vi "Receiver_Example.vi"() -> ()   [LabVIEW 2014]
panel:
  out "created new?":bool
  out "XY Graph":cdb[](graph)
  out "Modulation parameter":T1
  out "string 2":string
  out "SIG valid?":bool
  out "Frequency offset":dbl
  in  "stop":bool
  out "USRP CoercedParamters":T2={"coerced IQ rate"=100000.0, "coerced carrier frequency"=100000.0, "coerced gain"=0.0} {"coerced gain" format="%#_6f"; "coerced carrier frequency" format="%#_6p"; "coerced IQ rate" format="%#_6p"}
  out "error out":errorcluster
  in  "Trigger level":dbl=0.005 format="%f"
  in  "error in (no error)":errorcluster
  in  "USRP ControledParameters":T3={"active antenna"="RX2", "gain"=20.0, "carrier frequency"=5800000000.0, "IQ rate"=2000000.0} {"IQ rate" format="%#_6p"; "carrier frequency" format="%#_6p"; "gain" format="%#_6f"}
  in  "device names":refnum<k15>="NI2900"
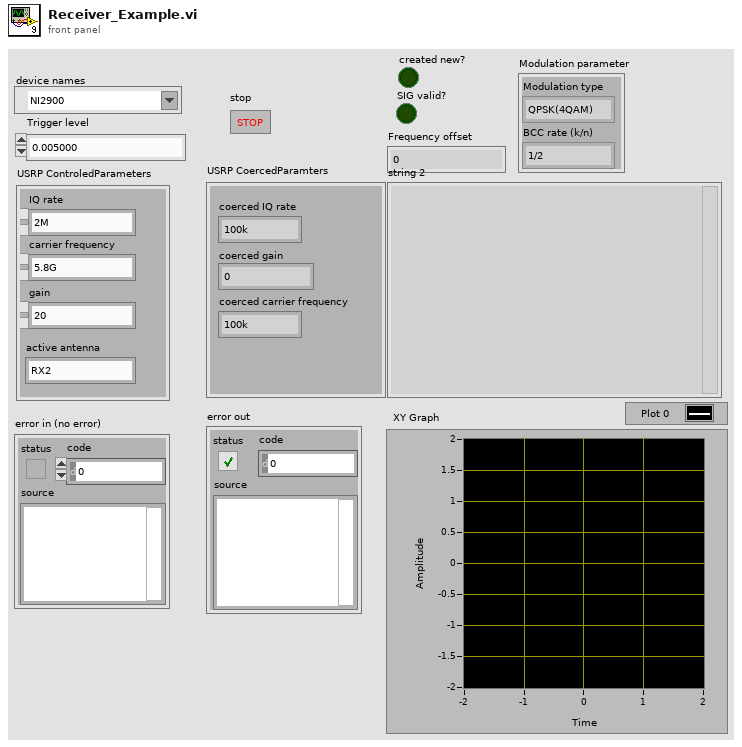
[diagram p1: front panel]
types:
  T1 = cluster{"Modulation type":enum16{"QPSK(4QAM)", "64QAM", "16QAM", "BPSK"}, "BCC rate (k/n)":enum16{"1/2", "2/3", "3/4"}}
  T2 = cluster{"coerced IQ rate":dbl, "coerced carrier frequency":dbl, "coerced gain":dbl}
  T3 = cluster{"active antenna":string, "gain":dbl, "carrier frequency":dbl, "IQ rate":dbl}
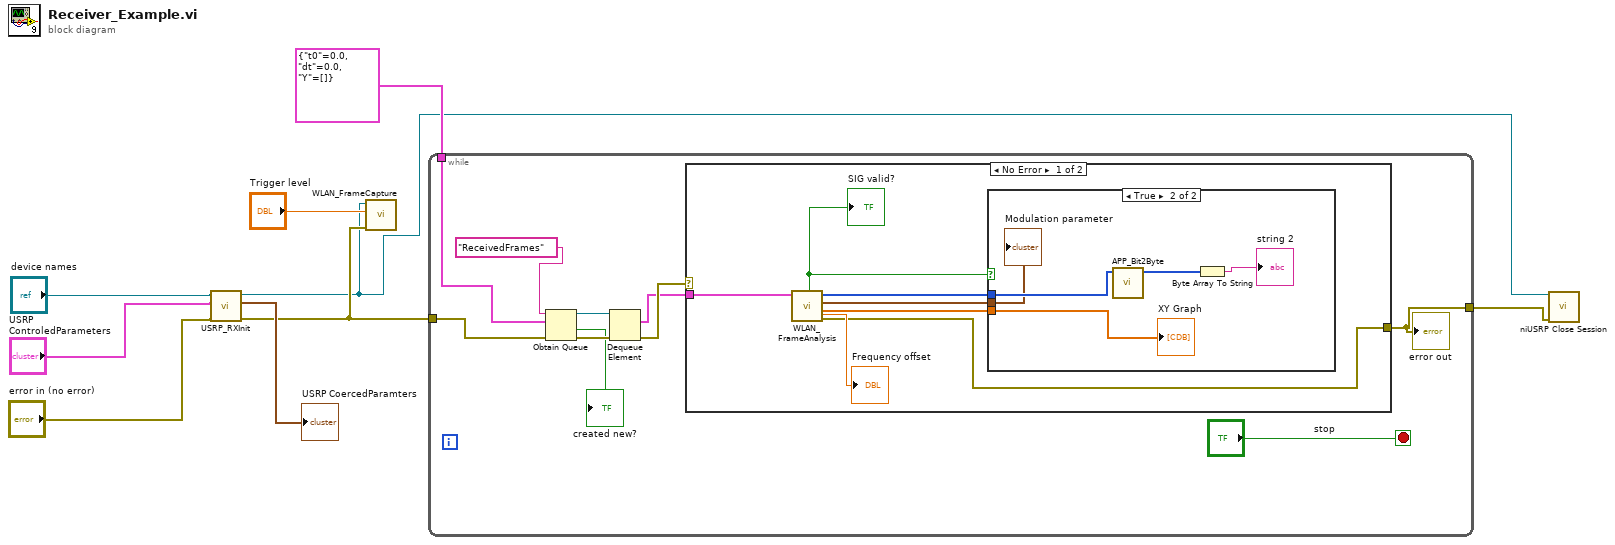
[diagram p0: block diagram]
diagram:
  n1 = call "USRP_RXInit.vi"("device names"="device names", "USRP ControledParameters"="USRP ControledParameters", "error in (no error)"="error in (no error)") -> ("session handle out"=w1:refnum<k15>, "USRP CoercedParamters"=→"USRP CoercedParamters":T2, "error out"=w5:errorcluster)  [unwired: 5 in]
  n2 = call "WLAN_FrameCapture.vi"("error in (no error)"=w5, "Trigger level"="Trigger level", "session handle"=w1) -> ()  [unwired: 8 in]
  n3 = while {
    tunnel: w5 -> [w17]
    tunnel: cluster{"t0":dbl, "dt":dbl, "Y":cdb[]} {"t0"=0.0, "dt"=0.0, "Y"=[]} ("data") -> [w18]
    tunnel: [w10] -> w2
    stop <- "stop" stop-if-true
    n4 = Obtain Queue(name (unnamed)="ReceivedFrames", element data type=w18, error in (no error)=w17) -> (queue out=w16:refnum<queue>, created new?=→"created new?":bool, error out=w13:errorcluster)  [unwired: 2 in]
    n5 = Dequeue Element(queue=w16, error in (no error)=w13) -> (element=w14:cluster{"t0":dbl, "dt":dbl, "Y":cdb[]}, error out=w15:errorcluster)  [unwired: 1 in, 2 out]
    n6 = case shown="No Error" w15 {
      selector: w15 -> [_ w32]
      tunnel: w14 -> [w20 _]
      tunnel: [w21 w32] -> w10
      frame No Error {
        n7 = call "WLAN_FrameAnalysis.vi"("input cluster"=w20) -> ("error out"=w21:errorcluster, "Constellation"=w23:cdb[], "Modulation parameter"=w22:T1, "output bits"=w24:i8[], "Frequency offset"=→"Frequency offset":dbl, "SIG valid?"=w25:bool)  [unwired: 5 in]
        "SIG valid?" <- w25
        n8 = case shown="True" w25 {
          tunnel: w24 -> [_ w31]
          tunnel: w23 -> [_ w29]
          tunnel: w22 -> [_ w30]
          frame False {
          }
          frame True {
            n9 = call "APP_Bit2Byte.vi"("input bit stream"=w31) -> ("output byte stream"=w27:u8[])  [unwired: 10 in]
            n10 = Byte Array To String(unsigned byte array=w27) -> (string=→"string 2":string)
            "Modulation parameter" <- w30
            "XY Graph" <- w29
          }
        }
      }
      frame Error {
      }
    }
    "error out" <- w10
  }
  n11 = call <instrlib>:"niUSRP Close Session.vi"("session handle"=w1, "error in (no error)"=w2) -> ()  [unwired: 13 in, 1 out]
